vi "List Map Providers.vi"(11 "InitProviders":string caption="ReqProvider") -> (1 "IdxInitPrvd":string, 2 "SelProvider":refnum<k24>, 3 "cmbProviders":cluster{"Name":string, string}[](array[cluster]), 5 "arrRefProviders":refnum<k24>[](array[refnum]), 7 "arr1DProviders":string[](array[string]))   [LabVIEW 2021, in "NMEA_GPS Ublox M8N.lvlib"]
uses:
  D:/My Projects/Ava Sanjesh Project/VI/GPS uBlox M8N Read/With GMap1.7.0/Data/GMap.NET.Core.dll
  Data/GMap.NET.Core.dll
  NMEA_GPS Ublox M8N.lvlib
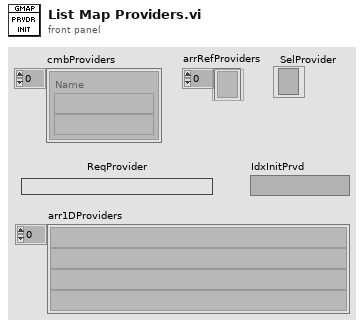
[diagram p1: front panel]
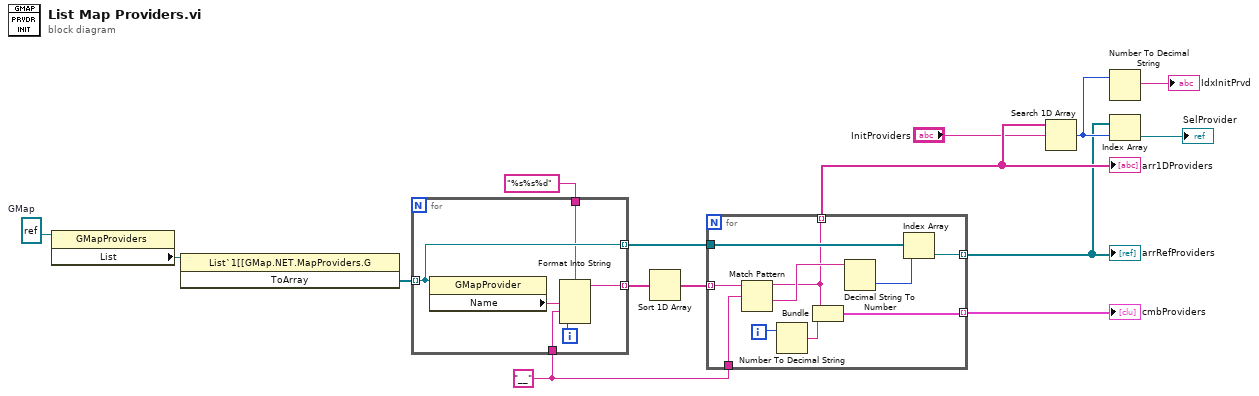
[diagram p0: block diagram]
diagram:
  w9 = "__" ("regular expression")
  w1 = refnum<k24> refnum  # GMap
  n1 = property class="GMapProviders"(reference=w1) -> ("List"=w13:refnum<k24>)  [unwired: 1 in, 2 out]
  n2 = invoke class="List`1[[GMap.NET.MapProviders.G" method="ToArray"(reference=w13) -> ("ToArray"=w14:refnum<k24>[])  [unwired: 2 in, 2 out]
  n3 = for {
    tunnel: w14 -> [w20] mode=indexing
    tunnel: [w21] -> w11 mode=indexing
    tunnel: [w20] -> w12 mode=indexing
    tunnel: "%s%s%d" ("format string") -> [w18]
    tunnel: w9 -> [w16]
    i -> [w17]
    n4 = property class="GMapProvider"(reference=w20) -> ("Name"=w19:string)  [unwired: 1 in, 2 out]
    n5 = Format Into String(format string=w18, w19, w16, w17) -> (resulting string=w21:string)  [unwired: 2 in, 1 out]
  }
  n6 = Sort 1D Array(array=w11) -> (sorted array=w8:string[])
  n7 = for {
    tunnel: w8 -> [w28] mode=indexing
    tunnel: [w29] -> w15 mode=indexing
    tunnel: w12 -> [w26]
    tunnel: [w24] -> w4 mode=indexing
    tunnel: w9 -> [w23]
    tunnel: [w22] -> w7 mode=indexing
    i -> [w30]
    n8 = Match Pattern(string=w28, regular expression=w23) -> (before substring=w22:string, after substring=w27:string)  [unwired: 1 in, 2 out]
    n9 = Number To Decimal String(number=w30) -> (decimal integer string=w31:string)  [unwired: 1 in]
    n10 = Bundle(w22, w31) -> (w29:cluster{string, string})  [unwired: 1 in]
    n11 = Decimal String To Number(string=w27) -> (number=w25:i32)  [unwired: 2 in, 1 out]
    n12 = Index Array(array=w26, index=w25) -> (element=w24:refnum<k24>)
  }
  "cmbProviders" <- w15
  "arrRefProviders" <- w4
  "arr1DProviders" <- w7
  n13 = Search 1D Array(1D array=w7, element="InitProviders") -> (index of element=w5:i32)  [unwired: 1 in]
  n14 = Number To Decimal String(number=w5) -> (decimal integer string=→"IdxInitPrvd":string)  [unwired: 1 in]
  n15 = Index Array(array=w4, index=w5) -> (element=→"SelProvider":refnum<k24>)
